vi "View AI param short scada.vi"(7 "ActivateAIView":bool, 8 "AINames":string[][](array[string]), 10 "AI_State":T3[](array[typedef]), 11 "AITable":dbl[](array[numeric]) format="%#.0f") -> (2 "Reread out":bool, 3 "This VI":refnum<vi>)   [LabVIEW 2019, in "Inputs.lvlib"]
uses:
  Ctl/Parameter State.ctl
  Ctl/AI.ctl
  Ctl/AI short.ctl
  Database/Progress.vi
  Inputs.lvlib
  Database/PostgreSQL.lvlib
  Logik/Logik.lvlib
panel:
  out "AI_9 2":dbl format="%#.1f"
  out "AI_10 2":dbl format="%#.1f"
  out "AI_5 2":dbl format="%#.1f"
  out "AI_6 2":dbl format="%#.1f"
  out "AI_7 2":dbl format="%#.1f"
  out "AI_8 2":dbl format="%#.1f"
  out "AI_3 2":dbl format="%#.1f"
  out "AI_4 2":dbl format="%#.1f"
  out "AI_2 2":dbl format="%#.1f"
  out "AI_1 2":dbl format="%#.1f"
  in  "AIP":T1
  out "AI progress":i32(slide) scale=0.0..100.0
  in  "Reread":bool
  in  "n_elem":i32(c297)
  out "units":string[](array[string])
  out "AI_9":dbl format="%#.1f"
  out "AI_10":dbl format="%#.1f"
  out "AI_5":dbl format="%#.1f"
  out "AI_6":dbl format="%#.1f"
  out "AI_7":dbl format="%#.1f"
  out "AI_8":dbl format="%#.1f"
  out "AI_3":dbl format="%#.1f"
  out "AI_4":dbl format="%#.1f"
  out "AI_2":dbl format="%#.1f"
  out "AI_1":dbl format="%#.1f"
  out "n param":i32
  out "Names":string[](array[string])=["температура нагревателя", "температура газа после ступени", "температура нагревателя", "температура нагревателя", "температура нагревателя", "температура газа после ступени", "давление газа перед нагревателем", "расход охлаждающей воды", "температура на входе", "температура на выходе", "регулятор расхода азота/тех газа", "давление охлаждающей воды на входе в теплообменник", "давление газа перед дозатором", "ток нагревателя", "температура нагревателя", "регулятор расхода азота/водорода (метана)", "давление газа перед дозатором", "регулятор расхода водорода (метана)", "регулятор природного газа", "дозатор жидкостный", "температура газа на входе в смеситель", "температура стенки смесителя 100 мм", "температура стенки смесителя 200 мм", "температура стенки смесителя на вводе CH4"]
  out "fcode":string[](array[string])=["H1.EB2.1.BT1", "H1.EB2.1.BT3", "H1.EB2.21.BT1", "H1.EB2.22.BT1", "H1.EB2.23.BT1", "H1.EB2.2.BT3", "H1.EB2.BP1", "H1.EB2.EP1.BF1", "H1.EB2.EP1.BT1", "H1.EB2.EP1.BT2", "H1.EB2.QN1", "H1.EP.BP1", "H1.GM2.1.BP1", "H1.GM2.1.HT1.BC1", "H1.GM2.1.HT1.BT1", "H1.GM2.1.QN1", "H1.GM2.2.BP1", "H1.GM2.2.QN1", "H1.GM2.2.QN2", "H1.GM2.2.QN3", "H1.HW2.BT1", "H1.HW2.BT2", "H1.HW2.BT3", "H1.HW2.BT4"]
  out "Parameters table":dbl[][](array[numeric])=[[1.0, 0.0, 1000.0, 2.0, 0.0, 0.0, 2.0, 20.0, 100.0, nan, 250.0, 250.0, 2.0, 1.0, 10.0, 0.0, 65535.0, 0.0, 250.0, 1.0, 4.0], [1.0, 0.0, 1000.0, 2.0, 0.0, 0.0, 2.0, 20.0, 150.0, nan, 250.0, 250.0, 2.0, 1.0, 11.0, 0.0, 65535.0, 0.0, 250.0, 0.0, 4.0], [1.0, 0.0, 1000.0, 2.0, 0.0, 0.0, 2.0, 3.0, 7.0, 8.0, 10.0, 10.0, 2.0, 0.1, 1.0, 0.0, 65535.0, 0.0, 10.0, 0.0, 2.0], [1.0, 0.0, 1000.0, 2.0, 0.0, 0.0, 1.5, 2.5, 6.0, 7.0, 10.0, 10.0, 2.0, 0.1, 2.0, 0.0, 65535.0, 0.0, 10.0, 0.0, 3.0], [1.0, 0.0, 1000.0, 2.0, 0.0, 0.0, 2.0, 2.5, 6.0, 7.0, 10.0, 10.0, 2.0, 0.1, 3.0, 0.0, 65535.0, 0.0, 10.0, 1.0, 2.0], [1.0, 0.0, 1000.0, 2.0, 0.0, 0.0, 1.5, 2.0, 4.0, 5.0, 10.0, 10.0, 2.0, 0.1, 4.0, 0.0, 65535.0, 0.0, 10.0, 1.0, 3.0], [1.0, 0.0, 1000.0, 2.0, 0.0, 0.0, 3.0, 4.0, 8.0, 9.0, 10.0, 10.0, 2.0, 0.1, 5.0, 0.0, 65535.0, 0.0, 100.0, 1.0, 7.0], [1.0, 0.0, 1000.0, 2.0, 0.0, 0.0, 4.0, 8.0, nan, nan, 100.0, 100.0, 2.0, 1.0, 6.0, 0.0, 65535.0, 0.0, 100.0, 0.0, 0.0], [1.0, 0.0, 1000.0, 2.0, 0.0, 0.0, nan, nan, nan, nan, 100.0, 100.0, 2.0, 1.0, 7.0, 0.0, 65535.0, 0.0, 100.0, 0.0, 1.0], [1.0, 0.0, 1000.0, 2.0, 0.0, 0.0, nan, nan, nan, nan, 100.0, 100.0, 2.0, 1.0, 8.0, 0.0, 65535.0, 0.0, 100.0, 1.0, 0.0], [1.0, 0.0, 1000.0, 2.0, 0.0, 0.0, 10.0, 15.0, 45.0, 50.0, 100.0, 100.0, 2.0, 1.0, 9.0, 0.0, 65535.0, 0.0, 100.0, 1.0, 1.0]]
  # "time_const"
  # "0%"
  # "LL"
  # "L"
  # "OK"
  # "H"
  # "HH"
  # "100 %"
  # "d"
  # "Analog parameters"
  # "Description of analog parameters"
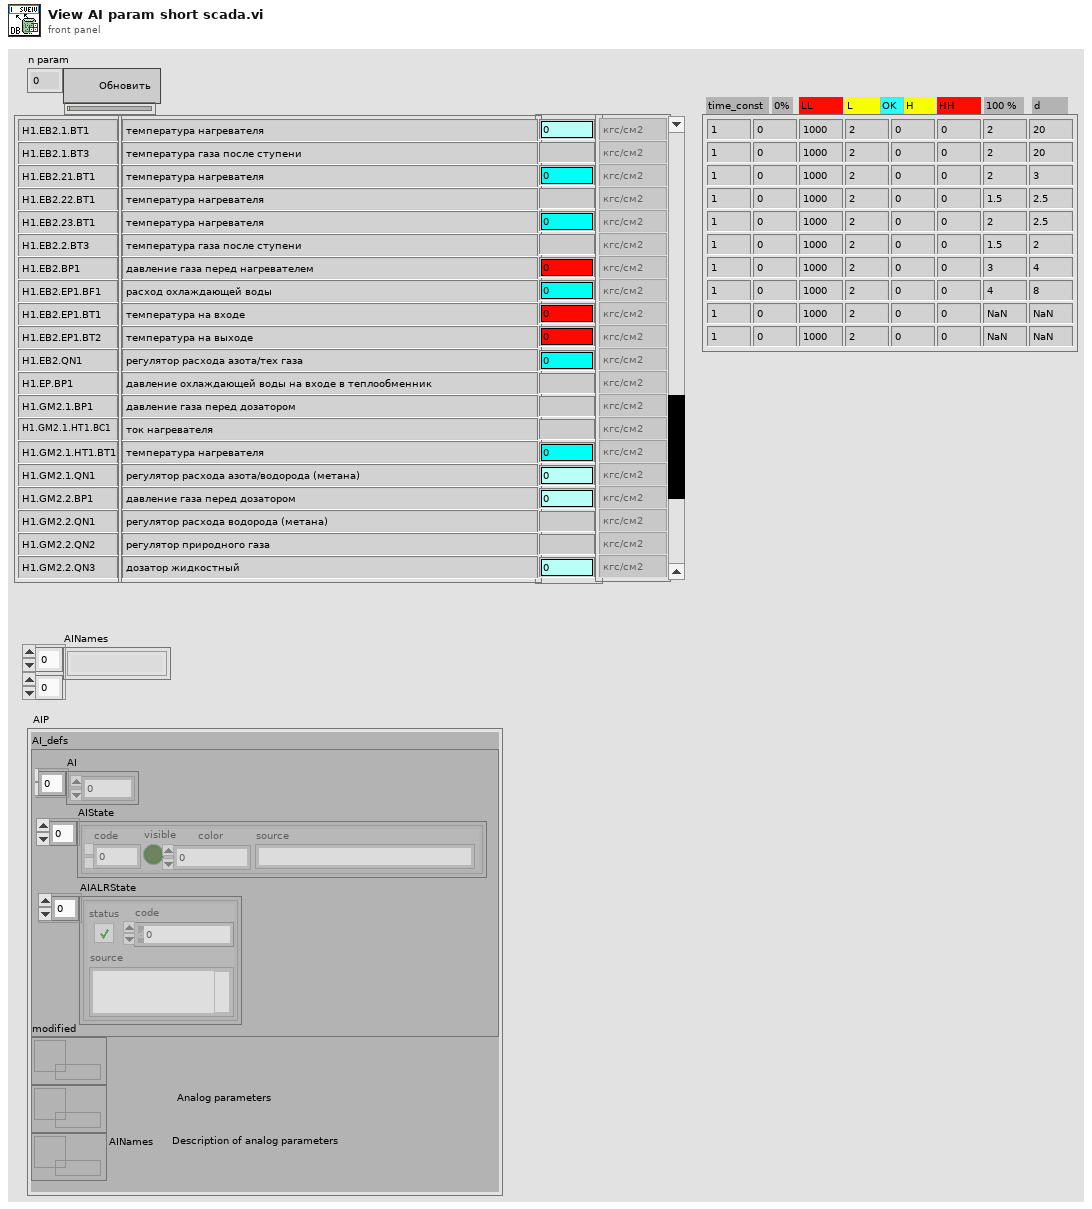
[diagram p1: front panel]
types:
  T1 = typedef "Inputs.lvlib/AI.ctl" = cluster{"AI_defs":T2, "modified":refnum<data-value>, "AIP":refnum<data-value>, "AINames":refnum<data-value>}
  T2 = typedef "Inputs.lvlib/AI short.ctl" = cluster{"AI":dbl[], "AIState":T3[], "AIALRState":errorcluster[]}
  T3 = typedef "Inputs.lvlib/Parameter State.ctl" = cluster{"code":i32, "visible":bool, "color":u32, "source":string}
  T4 = enum32{"Invalid", "Standard", "Closed", "Hidden", "Minimized", "Maximized"}
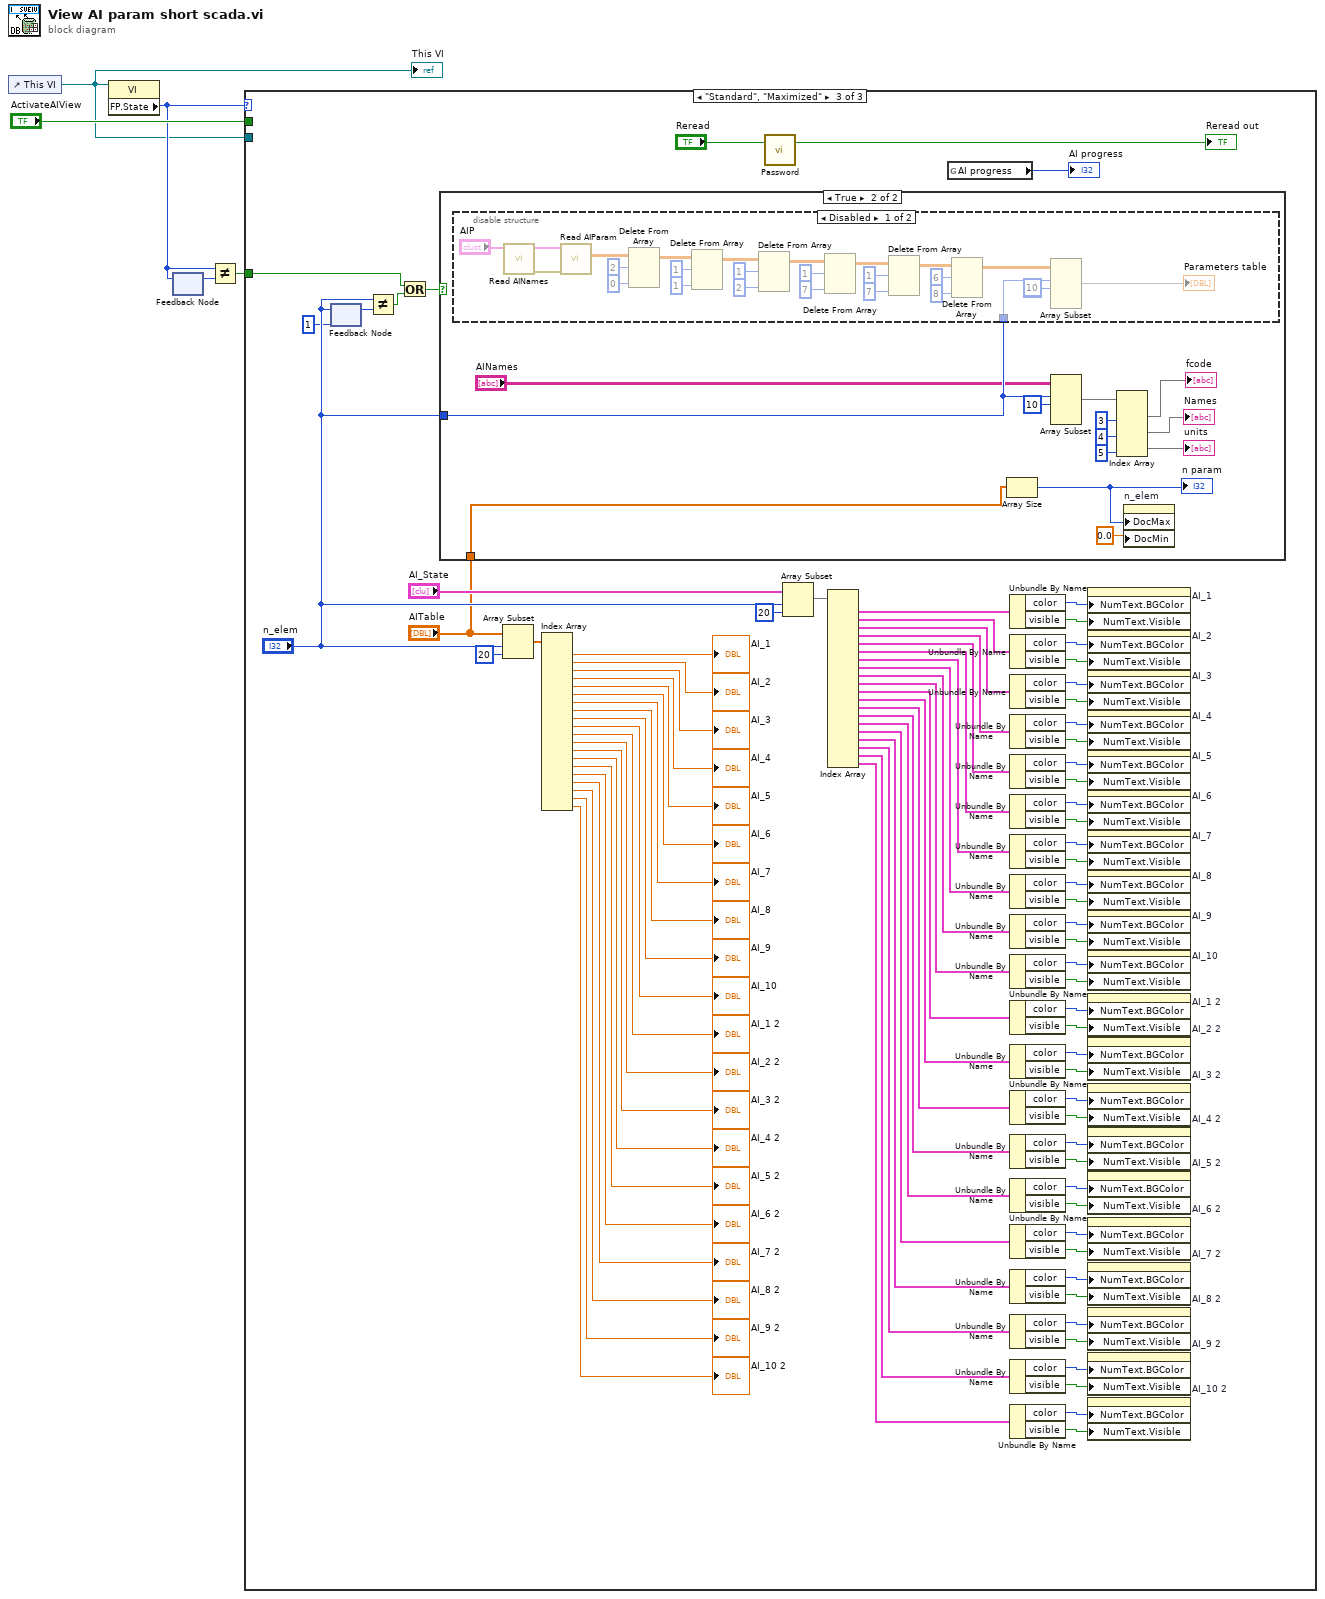
[diagram p0: block diagram]
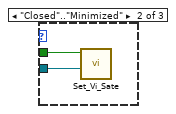
[diagram p3: hidden frame]
diagram:
  n1 = control-ref of="This VI"() -> (w1:refnum<vi>)
  "This VI" <- w1
  n2 = property class="VI"(reference=w1) -> ("FP.State"=w3:T4)  [unwired: 1 in, 2 out]
  n3 = feedback #1() -> (w4:T4)  [unwired: 1 in]
  n4 = feedback-in #1(w3) -> ()
  n5 = Not Equal?(x=w3, y=w4) -> (x != y?=w2:bool)
  n6 = case shown="\"Standard\", \"Maximized\"" w3 {
    tunnel: "ActivateAIView" -> [_ w6 _]
    tunnel: w1 -> [_ w7 _]
    tunnel: w2 -> [_ _ w50]
    frame "Invalid", Default {
    }
    frame "Closed".."Minimized" {
      n7 = call "Set_Vi_Sate.vi"("VI"=w7, "Activate (F)"=w6) -> ()  [unwired: 9 in, 1 out]
    }
    frame "Standard", "Maximized" {
      n8 = feedback #2(1 ("n_elem")) -> (w54:i32)
      n9 = feedback-in #2("n_elem") -> ()
      n10 = Not Equal?(x="n_elem", y=w54) -> (x != y?=w52:bool)
      n11 = Or(x=w50, y=w52) -> (x .or. y?=w51:bool)
      n12 = case shown="True" w51 {
        tunnel: "n_elem" -> [_ w112]
        tunnel: "AITable" -> [_ w104]
        frame False {
        }
        frame True {
          n13 = disable-structure shown="Disabled" {
            disable-tunnel: w112 -> [w138 _]
            frame Disabled {
              (unwired) 10 ("length")
              n14 = call "Read AINames.vi"("AI in"="AIP") -> ("error out"=w118:errorcluster, "AI out"=w116:T1)  [unwired: 8 in, 1 out]
              n15 = call "Read AIParam.vi"("error in (no error)"=w118, "AI in"=w116) -> ("AIParam"=w119:dbl[][])  [unwired: 7 in, 2 out]
              n16 = Delete From Array(array=w119, length=2, index (col)=0 ("disabled index (col)")) -> (array with subset deleted=w125:dbl[][])  [unwired: 1 in, 1 out]
              n17 = Delete From Array(array=w125, length=1, index (col)=1 ("disabled index (col)")) -> (array with subset deleted=w132:dbl[][])  [unwired: 1 in, 1 out]
              n18 = Delete From Array(array=w132, length=1, index (col)=2 ("disabled index (col)")) -> (array with subset deleted=w133:dbl[][])  [unwired: 1 in, 1 out]
              n19 = Delete From Array(array=w133, length=1, index (col)=7 ("disabled index (col)")) -> (array with subset deleted=w135:dbl[][])  [unwired: 1 in, 1 out]
              n20 = Delete From Array(array=w135, length=1, index (col)=7 ("disabled index (col)")) -> (array with subset deleted=w136:dbl[][])  [unwired: 1 in, 1 out]
              n21 = Delete From Array(array=w136, length=6, index (col)=8 ("disabled index (col)")) -> (array with subset deleted=w137:dbl[][])  [unwired: 1 in, 1 out]
              n22 = Array Subset(array=w137, index (row)=w138, length (row)=10 ("length")) -> (→"Parameters table":dbl[][])  [unwired: 2 in]
            }
            frame Enabled {
            }
          }
          n23 = Array Size(array=w104) -> (size(s)=w103:i32)
          "n param" <- w103
          n24 = Array Subset(array="AINames", index (row)=w112, length (row)=10 ("length")) -> (w115:string[][])  [unwired: 2 in]
          n25 = Index Array(array=w115, index (col) #1=3 ("disabled index (col)"), index (col) #2=4 ("disabled index (col)"), index (col) #3=5 ("index (col)")) -> (element #1=→"fcode":string[], element #2=→"Names":string[], element #3=→"units":string[])  [unwired: 3 in]
          n26 = property on="n_elem" class="Scroll (strict)"("DocMax"=w103, "DocMin"=0.0 ("Data Entry Limits:Minimum")) -> ()  [unwired: 2 in, 2 out]
        }
      }
      n27 = Array Subset(array="AITable", index="n_elem", length=20) -> (w91:dbl[])
      n28 = Index Array(array=w91) -> (element #1=→"AI_1":dbl, element #2=→"AI_2":dbl, element #3=→"AI_3":dbl, element #4=→"AI_4":dbl, element #5=→"AI_5":dbl, element #6=→"AI_6":dbl, element #7=→"AI_7":dbl, element #8=→"AI_8":dbl, element #9=→"AI_9":dbl, element #10=→"AI_10":dbl, element #11=→"AI_1 2":dbl, element #12=→"AI_2 2":dbl, element #13=→"AI_3 2":dbl, element #14=→"AI_4 2":dbl, element #15=→"AI_5 2":dbl, element #16=→"AI_6 2":dbl, element #17=→"AI_7 2":dbl, element #18=→"AI_8 2":dbl, element #19=→"AI_9 2":dbl, element #20=→"AI_10 2":dbl)  [unwired: 20 in]
      n29 = call "Password.vi"("ActivatePASSWView"="Reread") -> ("enable"=→"Reread out":bool)  [unwired: 1 in, 1 out]
      n30 = Array Subset(array="AI_State", index="n_elem", length=20) -> (w62:T3[])
      n31 = Index Array(array=w62) -> (element #1=w63:T3, element #2=w64:T3, element #3=w65:T3, element #4=w84:T3, element #5=w85:T3, element #6=w86:T3, element #7=w87:T3, element #8=w88:T3, element #9=w89:T3, element #10=w90:T3, element #11=w28:T3, element #12=w27:T3, element #13=w26:T3, element #14=w25:T3, element #15=w24:T3, element #16=w23:T3, element #17=w22:T3, element #18=w21:T3, element #19=w20:T3, element #20=w19:T3)  [unwired: 20 in]
      n32 = global read "Progress.vi" "AI progress"() -> (→"AI progress":i32)
      n33 = Unbundle By Name(w63) -> ("color"=w57:u32, "visible"=w58:bool)
      n34 = Unbundle By Name(w64) -> ("color"=w66:u32, "visible"=w67:bool)
      n35 = Unbundle By Name(w65) -> ("color"=w68:u32, "visible"=w69:bool)
      n36 = Unbundle By Name(w84) -> ("color"=w70:u32, "visible"=w71:bool)
      n37 = Unbundle By Name(w85) -> ("color"=w72:u32, "visible"=w73:bool)
      n38 = Unbundle By Name(w86) -> ("color"=w74:u32, "visible"=w75:bool)
      n39 = Unbundle By Name(w87) -> ("color"=w76:u32, "visible"=w77:bool)
      n40 = Unbundle By Name(w88) -> ("color"=w78:u32, "visible"=w79:bool)
      n41 = Unbundle By Name(w89) -> ("color"=w80:u32, "visible"=w81:bool)
      n42 = Unbundle By Name(w90) -> ("color"=w82:u32, "visible"=w83:bool)
      n43 = Unbundle By Name(w28) -> ("color"=w48:u32, "visible"=w47:bool)
      n44 = Unbundle By Name(w27) -> ("color"=w45:u32, "visible"=w46:bool)
      n45 = Unbundle By Name(w26) -> ("color"=w44:u32, "visible"=w43:bool)
      n46 = Unbundle By Name(w25) -> ("color"=w41:u32, "visible"=w42:bool)
      n47 = Unbundle By Name(w24) -> ("color"=w40:u32, "visible"=w39:bool)
      n48 = Unbundle By Name(w23) -> ("color"=w37:u32, "visible"=w38:bool)
      n49 = Unbundle By Name(w22) -> ("color"=w36:u32, "visible"=w35:bool)
      n50 = Unbundle By Name(w21) -> ("color"=w33:u32, "visible"=w34:bool)
      n51 = Unbundle By Name(w20) -> ("color"=w32:u32, "visible"=w31:bool)
      n52 = Unbundle By Name(w19) -> ("color"=w29:u32, "visible"=w30:bool)
      n53 = property on="AI_1" class="DigNum (strict)"("NumText.BGColor"=w57, "NumText.Visible"=w58) -> ()  [unwired: 2 in, 2 out]
      n54 = property on="AI_2" class="DigNum (strict)"("NumText.BGColor"=w66, "NumText.Visible"=w67) -> ()  [unwired: 2 in, 2 out]
      n55 = property on="AI_3" class="DigNum (strict)"("NumText.BGColor"=w68, "NumText.Visible"=w69) -> ()  [unwired: 2 in, 2 out]
      n56 = property on="AI_4" class="DigNum (strict)"("NumText.BGColor"=w70, "NumText.Visible"=w71) -> ()  [unwired: 2 in, 2 out]
      n57 = property on="AI_5" class="DigNum (strict)"("NumText.BGColor"=w72, "NumText.Visible"=w73) -> ()  [unwired: 2 in, 2 out]
      n58 = property on="AI_6" class="DigNum (strict)"("NumText.BGColor"=w74, "NumText.Visible"=w75) -> ()  [unwired: 2 in, 2 out]
      n59 = property on="AI_7" class="DigNum (strict)"("NumText.BGColor"=w76, "NumText.Visible"=w77) -> ()  [unwired: 2 in, 2 out]
      n60 = property on="AI_8" class="DigNum (strict)"("NumText.BGColor"=w78, "NumText.Visible"=w79) -> ()  [unwired: 2 in, 2 out]
      n61 = property on="AI_9" class="DigNum (strict)"("NumText.BGColor"=w80, "NumText.Visible"=w81) -> ()  [unwired: 2 in, 2 out]
      n62 = property on="AI_10" class="DigNum (strict)"("NumText.BGColor"=w82, "NumText.Visible"=w83) -> ()  [unwired: 2 in, 2 out]
      n63 = property on="AI_1 2" class="DigNum (strict)"("NumText.BGColor"=w48, "NumText.Visible"=w47) -> ()  [unwired: 2 in, 2 out]
      n64 = property on="AI_2 2" class="DigNum (strict)"("NumText.BGColor"=w45, "NumText.Visible"=w46) -> ()  [unwired: 2 in, 2 out]
      n65 = property on="AI_3 2" class="DigNum (strict)"("NumText.BGColor"=w44, "NumText.Visible"=w43) -> ()  [unwired: 2 in, 2 out]
      n66 = property on="AI_4 2" class="DigNum (strict)"("NumText.BGColor"=w41, "NumText.Visible"=w42) -> ()  [unwired: 2 in, 2 out]
      n67 = property on="AI_5 2" class="DigNum (strict)"("NumText.BGColor"=w40, "NumText.Visible"=w39) -> ()  [unwired: 2 in, 2 out]
      n68 = property on="AI_6 2" class="DigNum (strict)"("NumText.BGColor"=w37, "NumText.Visible"=w38) -> ()  [unwired: 2 in, 2 out]
      n69 = property on="AI_7 2" class="DigNum (strict)"("NumText.BGColor"=w36, "NumText.Visible"=w35) -> ()  [unwired: 2 in, 2 out]
      n70 = property on="AI_8 2" class="DigNum (strict)"("NumText.BGColor"=w33, "NumText.Visible"=w34) -> ()  [unwired: 2 in, 2 out]
      n71 = property on="AI_9 2" class="DigNum (strict)"("NumText.BGColor"=w32, "NumText.Visible"=w31) -> ()  [unwired: 2 in, 2 out]
      n72 = property on="AI_10 2" class="DigNum (strict)"("NumText.BGColor"=w29, "NumText.Visible"=w30) -> ()  [unwired: 2 in, 2 out]
    }
  }
